vi "HandleAlarms.vi"(0 "reference in":refnum<class "Sig_Digital.lvclass">, 11 "error in (no error)":errorcluster) -> (4 "reference out":refnum<class "Sig_Digital.lvclass">, 15 "error out":errorcluster)   [LabVIEW 2019, in "Sig_Digital.lvclass"]
uses:
  Sig_Digital.lvclass
  D:/GIT H4000/H4000/src/Proccess_class/Proccess.lvclass
  Sig_Digital.lvclass/Sig_Digital.ctl
  Proccess_class/Proccess.lvclass/Proccess.ctl
  Logger_class/EventCode.ctl
  Logger_class/Priority.ctl
  Logger_class/EventData.ctl
  Logger_class/Logger.lvclass
  Proccess_class/Proccess.lvclass
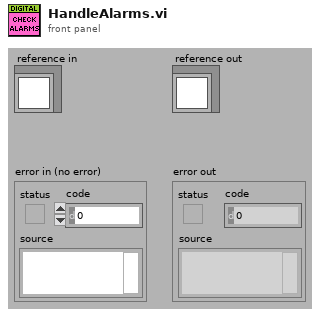
[diagram p1: front panel]
types:
  T1 = typedef "Logger.lvclass/EventCode.ctl" = enum16{"DI_EU_LO", "DI_EU_HI", "DIO_LO", "DIO_HI", "DI_RAW_LO", "DI_RAW_HI", "DO_LO", "DO_HI", "DA_OK", "DA_ALARM", "AA_HI", "AA_HIHI", "AA_LO", "AA_LOLO", "AA_OK", "CMD", "OUT_OF_RANGE_OK", "OUT_OF_RANGE_LO", "OUT_OF_RANGE_HI", "CONFIG", "DI_LO", "DI_HI"}
  T2 = typedef "Logger.lvclass/Priority.ctl" = enum16{"Alert", "Critical", "Error", "Warning", "Notice", "Informational", "Debug"}
  T3 = typedef "Logger.lvclass/EventData.ctl" = cluster{"obj_tag":string, "event_tag":string, "code":T1, "Priority":T2, "Value":dbl, "Description":string, "Time Stamp":timestamp}
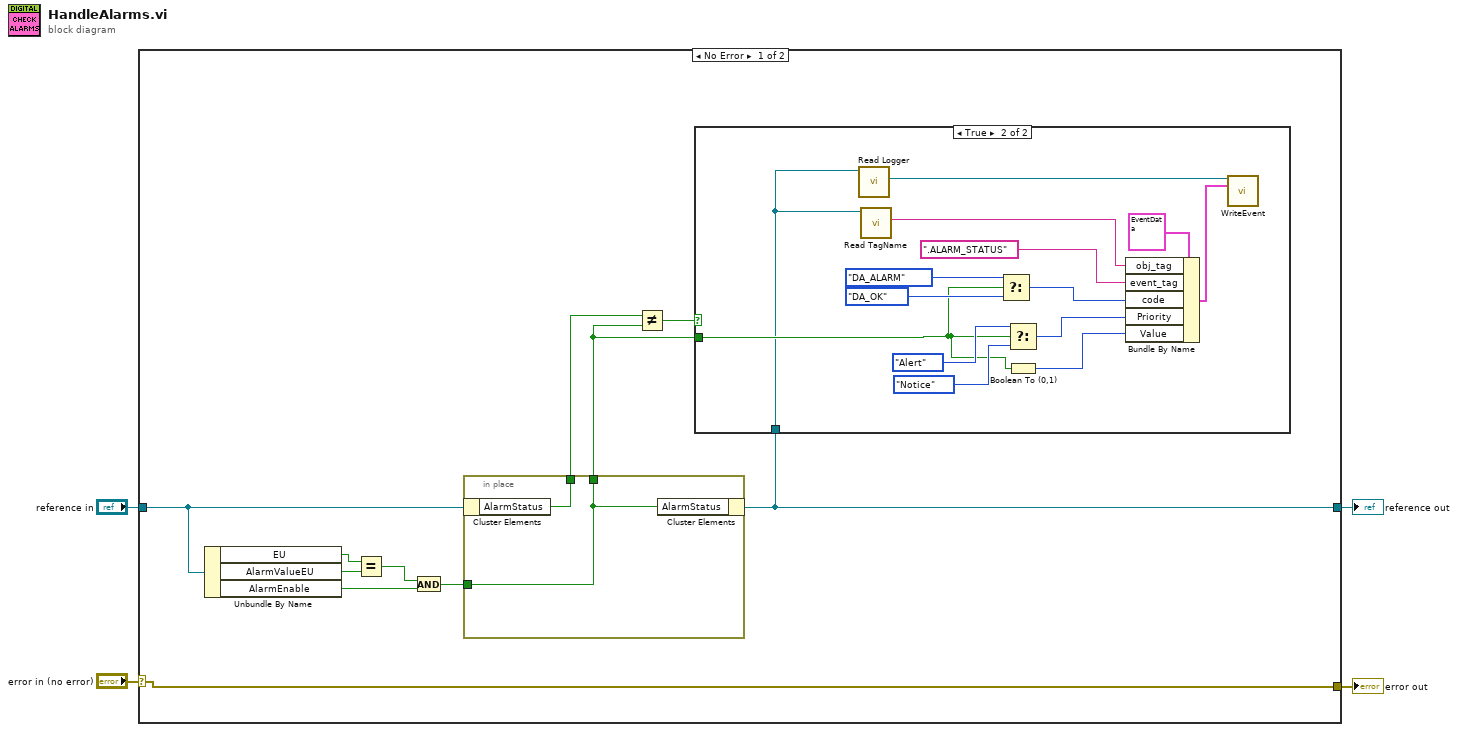
[diagram p0: block diagram]
diagram:
  n1 = case shown="No Error" "error in (no error)" {
    selector: "error in (no error)" -> [w14 w33]
    tunnel: [w14 w33] -> w3
    tunnel: [w5 w32] -> w1
    tunnel: "reference in" -> [w15 w32]
    frame No Error {
      n2 = Unbundle By Name(w15) -> ("EU"=w12:bool, "AlarmValueEU"=w11:bool, "AlarmEnable"=w9:bool)
      n3 = Equal?(x=w12, y=w11) -> (x = y?=w10:bool)
      n4 = And(x=w10, y=w9) -> (x .and. y?=w8:bool)
      n5 = in-place {
        in-place-border: w8 -> [w16]
        in-place-border: [w17] -> w7
        in-place-border: [w16] -> w6
        n6 = in-place-cluster #1(w15) -> ("AlarmStatus"=w17:bool)
        n7 = in-place-cluster #1("AlarmStatus"=w16) -> (w5:refnum<class "Sig_Digital.lvclass">)
      }
      n8 = Not Equal?(x=w7, y=w6) -> (x != y?=w13:bool)
      n9 = case shown="True" w13 {
        tunnel: w6 -> [_ w22]
        tunnel: w5 -> [_ w18]
        frame False {
        }
        frame True {
          n10 = call "Read Logger.vi"("Proccess in"=w18) -> ("Logger"=w19:refnum<class "Logger.lvclass">)  [unwired: 9 in, 1 out]
          n11 = call "Read TagName.vi"("Proccess in"=w18) -> ("TagName"=w20:string)  [unwired: 9 in, 1 out]
          n12 = Select(t=EventCode."DA_ALARM" ("Event"), s=w22, f=EventCode."DA_OK") -> (s? t:f=w24:T1)
          n13 = Select(t=Priority."Alert" ("Array"), s=w22, f=Priority."Notice") -> (s? t:f=w28:T2)
          n14 = Boolean To (0,1)(Boolean=w22) -> (0, 1=w21:i16)
          n15 = Bundle By Name(cluster=T3 {"obj_tag"="", "event_tag"="", "code"=enum."DI_RAW_LO", "Priority"=enum."Alert", "Value"=0.0, "Description"="", "Time Stamp"=timestamp(0 s since 1904-01-01)} ("Event"), "obj_tag"=w20, "event_tag"=".ALARM_STATUS" ("Event"), "code"=w24, "Priority"=w28, "Value"=w21) -> (w30:T3)
          n16 = call "WriteEvent.vi"("reference in"=w19, "Event"=w30) -> ()  [unwired: 12 in, 2 out]
        }
      }
    }
    frame Error {
    }
  }
  "error out" <- w3
  "reference out" <- w1
